vi "stop.vi"(8 "error in (no error)":errorcluster, 11 "Hamamatsu_C9100-13 in":refnum<class "Hamamatsu_C9100-13.lvclass">) -> (0 "error out":errorcluster, 3 "Hamamatsu_C9100-13 out":refnum<class "Hamamatsu_C9100-13.lvclass">)   [LabVIEW 2013, in "Hamamatsu_C9100-13.lvclass"]
uses:
  Hamamatsu_C9100-13.lvclass
  Hamamatsu_C9100-13.lvclass/Hamamatsu_C9100-13.ctl
  Camera.lvclass
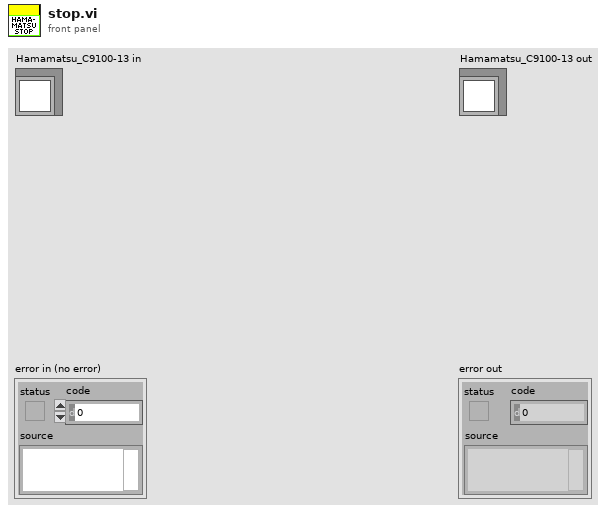
[diagram p1: front panel]
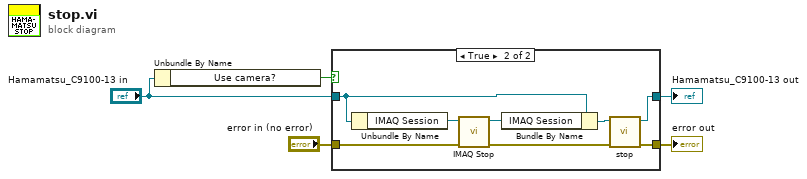
[diagram p0: block diagram]
diagram:
  n1 = Unbundle By Name("Hamamatsu_C9100-13 in") -> ("Use camera?"=w1:bool)
  n2 = case shown="True" w1 {
    tunnel: [w7 w15] -> w5
    tunnel: "error in (no error)" -> [w6 w14]
    tunnel: [w6 w13] -> w3
    tunnel: "Hamamatsu_C9100-13 in" -> [w7 w11]
    frame False {
    }
    frame True {
      n3 = Unbundle By Name(w11) -> ("IMAQ Session"=w12:refnum<k11>)
      n4 = call <vilib>:"IMAQ Stop.vi"("error in (no error)"=w14, "IMAQ Session In"=w12) -> ("error out"=w9:errorcluster, "IMAQ Session Out"=w8:refnum<k11>)  [unwired: 8 in]
      n5 = Bundle By Name(cluster=w11, "IMAQ Session"=w8) -> (w10:refnum<class "Hamamatsu_C9100-13.lvclass">)
      n6 = call-parent "stop.vi"("error in (no error)"=w9, "Camera in"=w10) -> ("error out"=w13:errorcluster, "Camera out"=w15:refnum<class "Hamamatsu_C9100-13.lvclass">)  [unwired: 8 in]
    }
  }
  "error out" <- w3
  "Hamamatsu_C9100-13 out" <- w5
